vi "Read DO Waveforms.vi"(8 "error in (no error)":errorcluster, 11 "SequencerConfig in":refnum<class "SequencerConfig.lvclass">) -> (0 "error out":errorcluster, 2 "DO Waveforms":digitalwaveform[](array[waveform]), 3 "SequencerConfig out":refnum<class "SequencerConfig.lvclass">)   [LabVIEW 2015, in "Sequencer.lvlib" / "SequencerConfig.lvclass"]
uses:
  SequencerConfig.lvclass
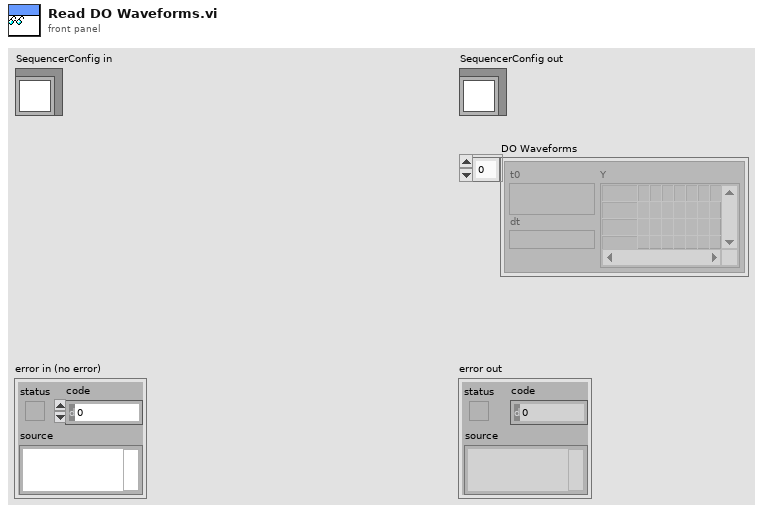
[diagram p1: front panel]
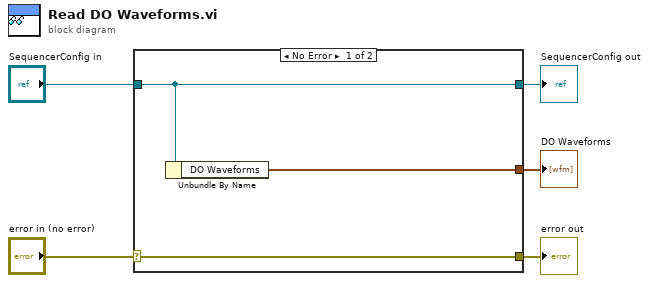
[diagram p0: block diagram]
diagram:
  n1 = case shown="No Error" "error in (no error)" {
    selector: "error in (no error)" -> [w8 w9]
    tunnel: [w8 w9] -> w4
    tunnel: [w7 w10] -> w2
    tunnel: "SequencerConfig in" -> [w7 w10]
    tunnel: [w6 _] -> w1
    frame No Error {
      n2 = Unbundle By Name(w7) -> ("DO Waveforms"=w6:digitalwaveform[])
    }
    frame Error {
    }
  }
  "error out" <- w4
  "SequencerConfig out" <- w2
  "DO Waveforms" <- w1
